vi "Configure Control Loop Response Power Analysis (Basic).vi"(6 "Output Channel (1: Channel 2)":i32(ring)=1 items=["Channel 1", "Channel 2", "Channel 3", "Channel 4"], 7 "Input Channel (0: Channel 1)":i32(ring) items=["Channel 1", "Channel 2", "Channel 3", "Channel 4"], 8 "error in (no error)":errorcluster, 9 "Trace (4: Gain and Phase)":i32(ring)=4 items=["None", "All", "Gain", "Phase", "Gain and Phase"], 10 "Point Number (10: 10)":i32(ring)=10 items=["10"=10, "20"=20, "30"=30, "40"=40, "50"=50, "60"=60, "70"=70, "80"=80, "90"=90, "100"=100], 11 "VISA resource name":refnum<visa-resource-name>) -> (0 "error out":errorcluster, 3 "VISA resource name out":refnum<visa-resource-name>)   [LabVIEW 2015, in "Agilent 2000 3000 X-Series.lvlib"]
doc: "Configures the basic setting for control loop response power analysis.\n\n<b>Note:</b>\n - This VI is applicable for 3000T, 3000G, 4000, 6000 X-Series."
uses:
  Agilent 2000 3000 X-Series.lvlib
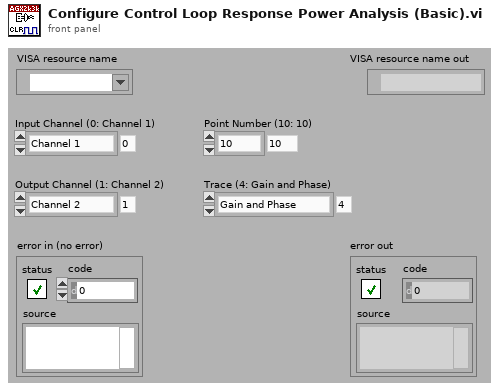
[diagram p1: front panel]
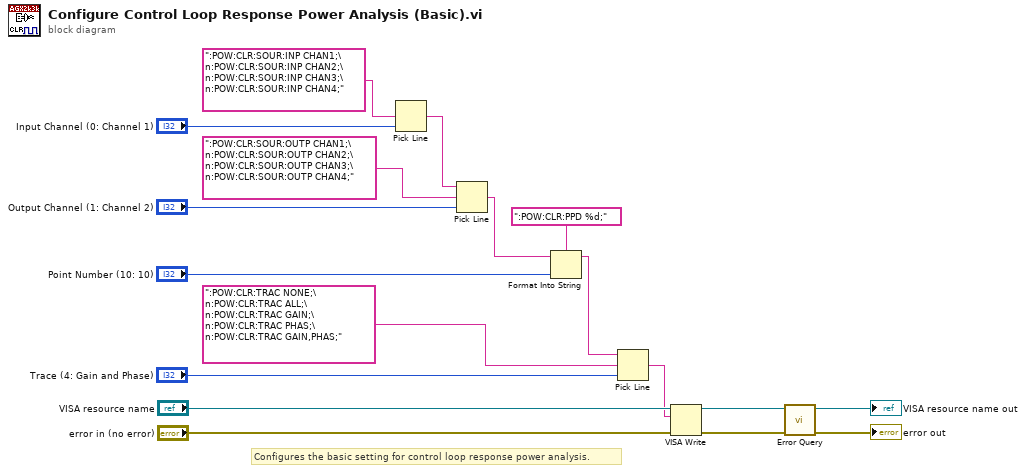
[diagram p0: block diagram]
diagram:
  # "Configures the basic setting for control loop response power analysis."
  n1 = Pick Line(multi-line string=":POW:CLR:SOUR:INP CHAN1;\n:POW:CLR:SOUR:INP CHAN2;\n:POW:CLR:SOUR:INP CHAN3;\n:POW:CLR:SOUR:INP CHAN4;", line index="Input Channel (0: Channel 1)") -> (output string=w9:string)  [unwired: 1 in]
  n2 = Pick Line(string ("")=w9, multi-line string=":POW:CLR:SOUR:OUTP CHAN1;\n:POW:CLR:SOUR:OUTP CHAN2;\n:POW:CLR:SOUR:OUTP CHAN3;\n:POW:CLR:SOUR:OUTP CHAN4;", line index="Output Channel (1: Channel 2)") -> (output string=w8:string)
  n3 = Format Into String(format string=":POW:CLR:PPD %d;", initial string=w8, "Point Number (10: 10)") -> (resulting string=w7:string)  [unwired: 1 in, 1 out]
  n4 = Pick Line(string ("")=w7, multi-line string=":POW:CLR:TRAC NONE;\n:POW:CLR:TRAC ALL;\n:POW:CLR:TRAC GAIN;\n:POW:CLR:TRAC PHAS;\n:POW:CLR:TRAC GAIN,PHAS;", line index="Trace (4: Gain and Phase)") -> (output string=w6:string)
  n5 = VISA Write(VISA resource name="VISA resource name", write buffer=w6, error in (no error)="error in (no error)") -> (VISA resource name out=w5:refnum<visa-resource-name>, error out=w3:errorcluster)  [unwired: 1 out]
  n6 = call "Error Query.vi"("error in (no error)"=w3, "VISA resource name"=w5) -> ("error out"=→"error out":errorcluster, "VISA resource name out"=→"VISA resource name out":refnum<visa-resource-name>)  [unwired: 6 in, 2 out]
